vi "Refresh Layout.vi"(8 "error in (no error)":errorcluster, 11 "2DArrayManager in":refnum<class "2DArrayManager.lvclass">) -> (0 "error out":errorcluster, 3 "2DArrayManager out":refnum<class "2DArrayManager.lvclass">)   [LabVIEW 2020, in "OOPanel.lvlib" / "2DArrayManager.lvclass"]
uses:
  2DArrayManager.lvclass
  2DArrayManager.lvclass/2DArrayManager.ctl
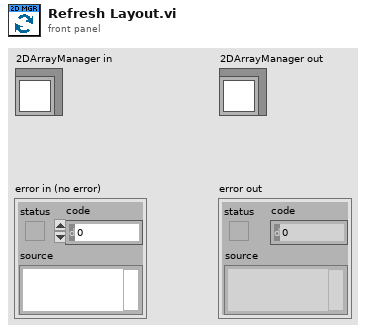
[diagram p1: front panel]
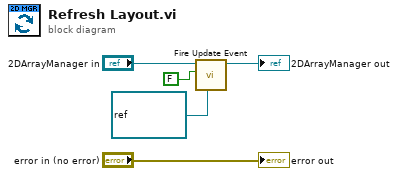
[diagram p0: block diagram]
diagram:
  n1 = call "Fire Update Event.vi"("Sync Response"=refnum<notifier> refnum, "Synced"=FALSE, "2DArrayManager in"="2DArrayManager in") -> ("2DArrayManager out"=→"2DArrayManager out":refnum<class "2DArrayManager.lvclass">)  [unwired: 7 in, 1 out]
  "error out" <- "error in (no error)"
